vi "Run Tests.vi"(8 "error in (no error)":errorcluster, 10 "Filter":T1, 11 "Execution UI in":refnum<class "Execution UI.lvclass">) -> (0 "error out":errorcluster, 3 "Execution UI out":refnum<class "Execution UI.lvclass">)   [LabVIEW 2020, in "Execution UI.lvclass"]
uses:
  Execution UI.lvclass
  Result Model/Tree Item Filter.ctl
  C:/git/astemes-lunit/source/User Interface/Process/Process.lvclass
  Execution UI.lvclass/Execution UI.ctl
  Process/Process.lvclass/Process.ctl
  Process/Process.lvclass
  Result Model by Reference/Result Model by Reference.lvclass
  Result Model/Result Model.lvclass
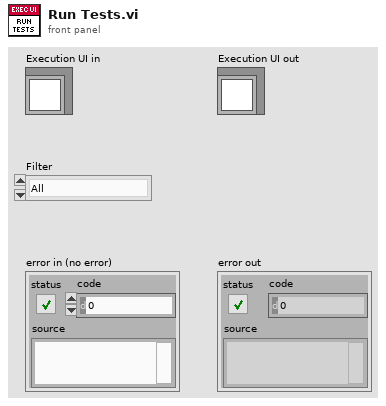
[diagram p1: front panel]
types:
  T1 = typedef "Result Model.lvclass/Tree Item Filter.ctl" = enum16{"All", "Only Fails", "Fails or else Not Executed"}
  T2 = cluster{"Left Cell String":string, "Child Text":string[], "Child Tag":string, "Item Indent":i32, "Child Only?":bool, "Glyph Index":i32}[]
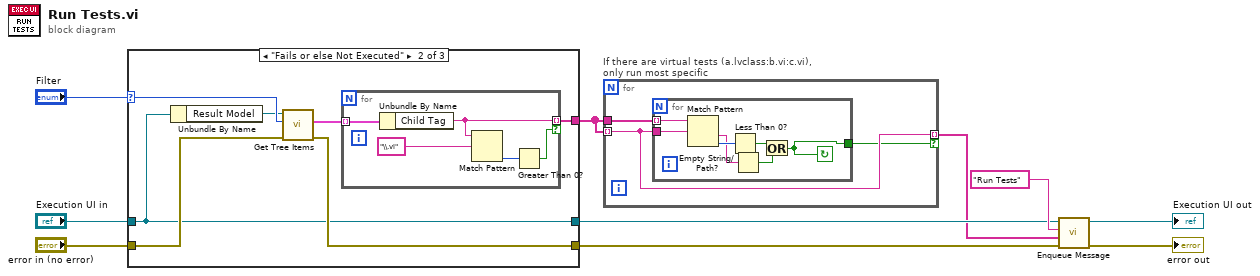
[diagram p0: block diagram]
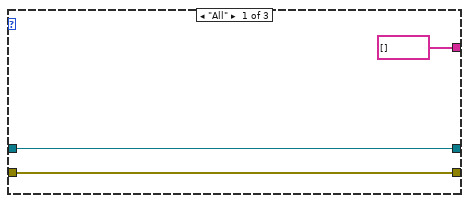
[diagram p2: hidden frame]
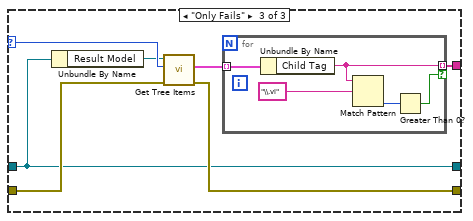
[diagram p3: hidden frame]
diagram:
  n1 = case shown="\"Fails or else Not Executed\"" "Filter" {
    selector: "Filter" -> [_ w18 w31]
    tunnel: [string[] [] w20 w26] -> w2
    tunnel: "error in (no error)" -> [w13 w17 w30]
    tunnel: [w13 w16 w29] -> w8
    tunnel: "Execution UI in" -> [w12 w14 w27]
    tunnel: [w12 w14 w27] -> w3
    frame "All" {
    }
    frame "Fails or else Not Executed" {
      n2 = Unbundle By Name(w14) -> ("Result Model"=w15:refnum<class "Result Model by Reference.lvclass">)
      n3 = call "Get Tree Items.vi"("error in (no error)"=w17, "Filter"=w18, "Result Model by Reference In"=w15) -> ("error out"=w16:errorcluster, "Tree Items"=w19:T2)  [unwired: 7 in]
      n4 = for {
        tunnel: w19 -> [w25] mode=indexing
        tunnel: [w23] -> w20 mode=indexing if=w21
        n5 = Unbundle By Name(w25) -> ("Child Tag"=w23:string)
        n6 = Match Pattern(string=w23, regular expression="\\.vi") -> (offset past match=w22:i32)  [unwired: 1 in, 3 out]
        n7 = Greater Than 0?(x=w22) -> (x > 0?=w21:bool)
      }
    }
    frame "Only Fails" {
      n8 = Unbundle By Name(w27) -> ("Result Model"=w28:refnum<class "Result Model by Reference.lvclass">)
      n9 = call "Get Tree Items.vi"("error in (no error)"=w30, "Filter"=w31, "Result Model by Reference In"=w28) -> ("error out"=w29:errorcluster, "Tree Items"=w32:T2)  [unwired: 7 in]
      n10 = for {
        tunnel: w32 -> [w37] mode=indexing
        tunnel: [w35] -> w26 mode=indexing if=w33
        n11 = Unbundle By Name(w37) -> ("Child Tag"=w35:string)
        n12 = Match Pattern(string=w35, regular expression="\\.vi") -> (offset past match=w34:i32)  [unwired: 1 in, 3 out]
        n13 = Greater Than 0?(x=w34) -> (x > 0?=w33:bool)
      }
    }
  }
  n14 = for "If there are virtual tests (a.lvclass:b.vi:c.vi), only run most specific" {
    tunnel: w2 -> [w40] mode=indexing
    tunnel: [w40] -> w1 mode=indexing if=w39
    tunnel: w2 -> [w38]
    n15 = for {
      tunnel: w38 -> [w47] mode=indexing
      tunnel: w40 -> [w46]
      tunnel: [w43] -> w39
      stop <- w43 continue-if-true
      n16 = Match Pattern(string=w47, regular expression=w46) -> (after substring=w42:string, offset past match=w45:i32)  [unwired: 1 in, 2 out]
      n17 = Less Than 0?(x=w45) -> (x < 0?=w44:bool)
      n18 = Empty String/Path?(string/path=w42) -> (empty?=w41:bool)
      n19 = Or(x=w44, y=w41) -> (x .or. y?=w43:bool)
    }
  }
  n20 = call "Enqueue Message.vi"("error in (no error)"=w8, "Message Data"=w1, "Message"="Run Tests", "Process In"=w3) -> ("error out"=→"error out":errorcluster, "Process Out"=→"Execution UI out":refnum<class "Execution UI.lvclass">)  [unwired: 6 in]
